vi "InitDriverControl.vi"   [LabVIEW 2023]
doc: "This VI initializes user interface devices."
uses:
  <vilib>/Rock Robotics/WPI/Joystick/WPI_JoystickDeviceEnum.ctl
  GlobalDriverStationCommands.vi
types:
  T1 = typedef "WPI_JoystickDeviceEnum.ctl" = enum16{"USB 0", "USB 1", "USB 2", "USB 3", "USB 4", "USB 5"}
  T2 = typedef "WPI_JoystickDevRef.ctl" = cluster{"Device":T1}
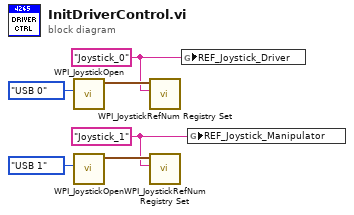
[diagram p0: block diagram]
diagram:
  w1 = "Joystick_1" ("Joystick_0")
  w2 = "Joystick_0" ("Joystick_0")
  n1 = call <vilib>:"WPI_JoystickOpen.vi"("JoystickDevice"=WPI_JoystickDeviceEnum."USB 0") -> ("JoystickDevRef"=w6:T2)  [unwired: 10 in]
  n2 = call <vilib>:"WPI_JoystickOpen.vi"("JoystickDevice"=WPI_JoystickDeviceEnum."USB 1") -> ("JoystickDevRef"=w4:T2)  [unwired: 10 in]
  n3 = call <vilib>:"WPI_JoystickRefNum Registry Set.vi"("refnum name"=w2, "JoystickDevRef"=w6) -> ()  [unwired: 8 in, 2 out]
  n4 = call <vilib>:"WPI_JoystickRefNum Registry Set.vi"("refnum name"=w1, "JoystickDevRef"=w4) -> ()  [unwired: 8 in, 2 out]
  n5 = global write "GlobalDriverStationCommands.vi" "REF_Joystick_Driver"(w2) -> ()
  n6 = global write "GlobalDriverStationCommands.vi" "REF_Joystick_Manipulator"(w1) -> ()
